vi "Copy Value.vi"(10 "From":refnum<class "Type.lvclass">, 11 "Text in":refnum<class "Text.lvclass">) -> (2 "error out":errorcluster, 3 "Text out":refnum<class "Text.lvclass">)   [LabVIEW 2020, in "Conditum.lvlib" / "Columns.lvlib" / "Text.lvclass"]
uses:
  Text.lvclass
  C:/dev/lv20CE/lv-conditum/Conditum/Columns/Type/Type.lvclass
  Type/Type.lvclass
  Text.lvclass/Text.ctl
  Type/Type.lvclass/Type.ctl
  Type/Clear NULL.vi
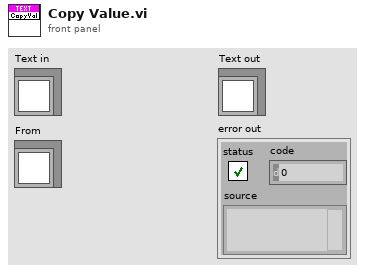
[diagram p1: front panel]
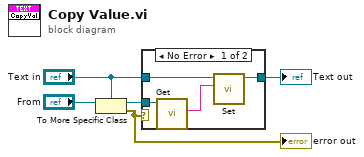
[diagram p0: block diagram]
diagram:
  n1 = To More Specific Class(target class="Text in", reference="From") -> (specific class reference=w5:refnum<class "Text.lvclass">, error out=w4:errorcluster)  [unwired: 1 in]
  "error out" <- w4
  n2 = case shown="No Error" w4 {
    tunnel: w5 -> [w9 _]
    tunnel: "Text in" -> [w7 w10]
    tunnel: [w6 w10] -> w3
    frame No Error {
      n3 = call "Get.vi"("Text in"=w9) -> ("Value"=w8:string)  [unwired: 10 in]
      n4 = call "Set.vi"("Value"=w8, "Text in"=w7) -> ("Text out"=w6:refnum<class "Text.lvclass">)  [unwired: 9 in]
    }
    frame Error {
    }
  }
  "Text out" <- w3
